vi "2020_day06.vi"() -> ()   [LabVIEW 2021]
panel:
  out "Task 2":i32
  out "Task 1":i32
  in  "Switch":bool caption="Ex. Data  vs.  User Data"
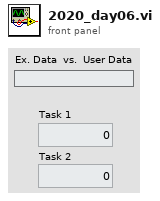
[diagram p1: front panel]
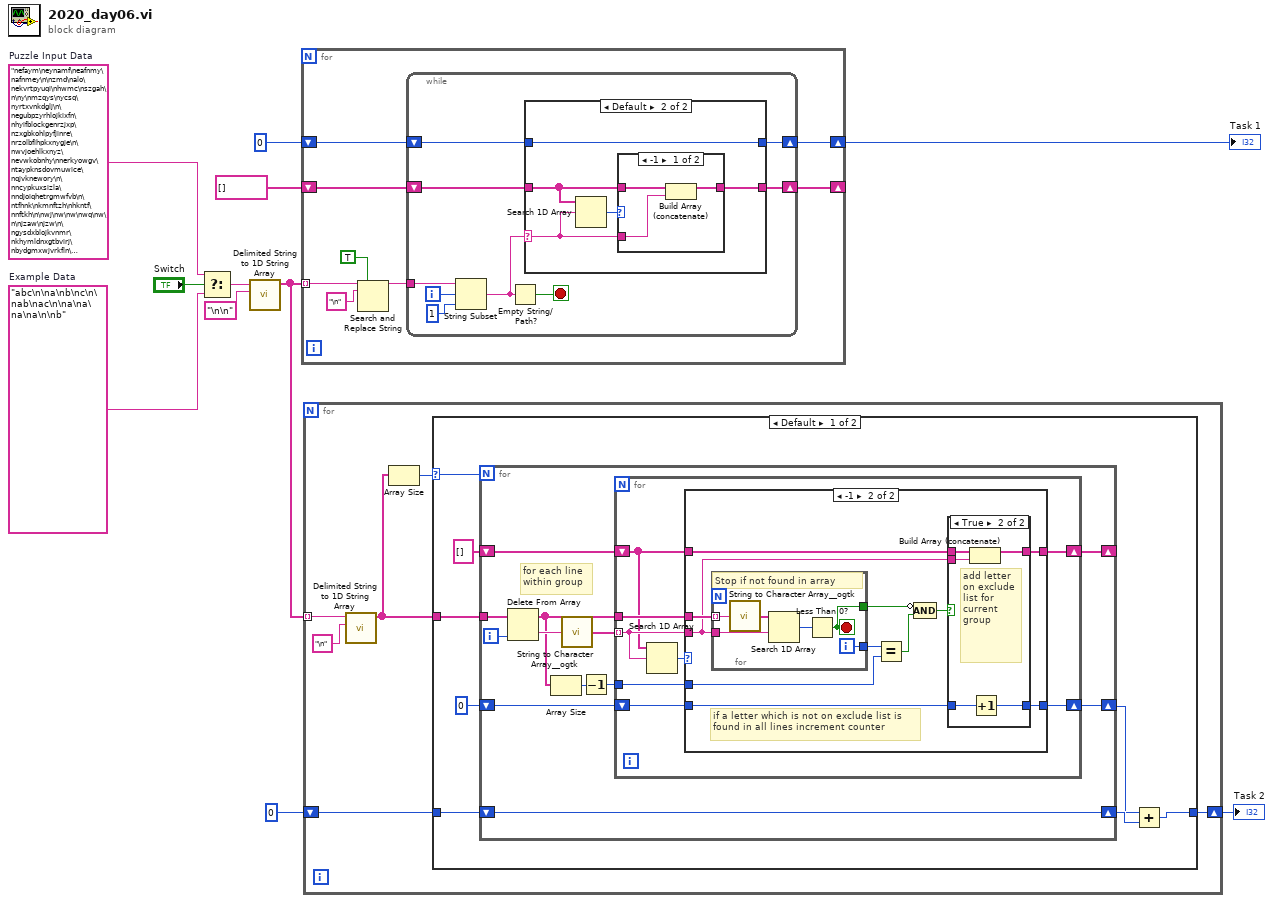
[diagram p0: block diagram]
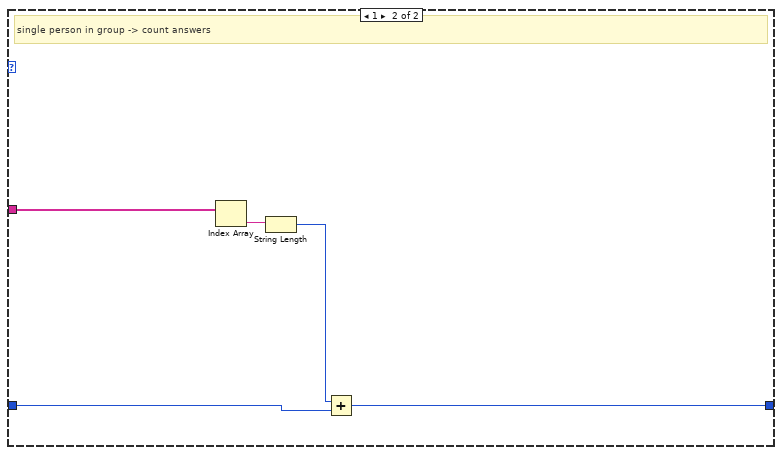
[diagram p4: hidden frame]
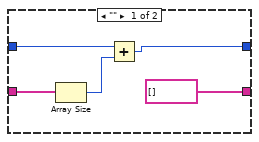
[diagram p5: hidden frame]
diagram:
  w9 = "nefaym\neynamf\neafnmy\nafnmey\n\nzmd\nalo\nekvrtpyuqi\nhwmc\nszgah\n\ny\nmzqys\nycsq\nyrtxvnkdglj\n\negubpzyrhlojkixfn\nhyifblockgenrzjxp\nzxgbkohlpyfjinre\nrzolbfihpkxnygje\n\nwvjoehlkxnyz\nevwkobnhy\nnerkyowgv\ntaypknsdovmuwice\nqjvknewory\n\nncypkuxsizla\nndjoiqhetrgmwfvb\n\ntfhnk\nkmnftzh\nhkntf\nnftkh\n\nwj\nw\nw\nwq\nw\n\njzaw\njzw\n\ngysdxblojkvnmr\nkhymldnxgtbvirj\nbydgmxwjvrkfln\nlykvumdnrxbjg\n\nxce\nxec\nxec\ncex\n\nlacbwdzjofymieug\nqpbhtnywsluirgjaxkfm\n\norzpamlyckgwhjidnq\nmyeqhzijgkdoxwprcvbt\ngzaocylrwkiumpfjqdh\ncqhzpwiyrmkdgjso\n\nd\nvd\nsgohd\n\nr\nr\n\nknyrgtba\ngatbyoknr\nakmgyntbr\narykgnbot\nanyrgbkt\n\niohn\ncoangpuj\non\nknqoi\ntoink\n\nhvramnt\ng..."  # Puzzle Input Data
  w10 = "abc\n\na\nb\nc\n\nab\nac\n\na\na\na\na\n\nb"  # Example Data
  n1 = Select(t=w9, s="Switch", f=w10) -> (s? t:f=w4:string)
  n2 = call <vilib>:"Delimited String to 1D String Array.vi"("delimiter"="\n\n", "delimited string"=w4) -> ("string array"=w1:string[])  [unwired: 9 in]
  n3 = for {
    tunnel: w1 -> [w15] mode=indexing
    shift-right: [w18] -> _
    shift-left: string[] [] ("array type (2D Dbl)") -> [w19]
    shift-right: [w16] -> w6
    shift-left: 0 -> [w17]
    n4 = Search and Replace String(replace all?=TRUE ("replace all? (F)"), input string=w15, search string="\n" ("delimiter")) -> (result string=w14:string)  [unwired: 5 in, 3 out]
    n5 = while {
      tunnel: w14 -> [w27]
      shift-right: [w22] -> w18
      shift-left: w19 -> [w28]
      shift-right: [w20] -> w16
      shift-left: w17 -> [w21]
      i -> [w26]
      stop <- w24 stop-if-true
      n6 = String Subset(string=w27, offset (0)=w26, length (rest)=1 ("length (rest)")) -> (substring=w23:string)
      n7 = Empty String/Path?(string/path=w23) -> (empty?=w24:bool)
      n8 = case shown="Default" w23 {
        selector: w23 -> [_ w35]
        tunnel: w28 -> [w30 w38]
        tunnel: [string[] [] ("array type (2D Dbl)") w37] -> w22
        tunnel: w21 -> [w32 w34]
        tunnel: [w31 w34] -> w20
        frame "" {
          n9 = Array Size(array=w30) -> (size(s)=w33:i32)
          n10 = Add(x=w32, y=w33) -> (x+y=w31:i32)
        }
        frame Default {
          n11 = Search 1D Array(1D array=w38, element=w35) -> (index of element=w36:i32)  [unwired: 1 in]
          n12 = case shown="-1" w36 {
            tunnel: w38 -> [w41 w42]
            tunnel: [w40 w42] -> w37
            tunnel: w35 -> [w39 _]
            frame -1 {
              n13 = Build Array (concatenate)(w41, w39) -> (w40:string[])
            }
            frame Default {
            }
          }
        }
      }
    }
  }
  "Task 1" <- w6
  n14 = for {
    tunnel: w1 -> [w48] mode=indexing
    shift-right: [w43] -> w2
    shift-left: 0 -> [w44]
    n15 = call <vilib>:"Delimited String to 1D String Array.vi"("delimiter"="\n", "delimited string"=w48) -> ("string array"=w45:string[])  [unwired: 9 in]
    n16 = Array Size(array=w45) -> (size(s)=w46:i32)
    n17 = case shown="Default" w46 {
      selector: w46 -> [w53 _]
      tunnel: w45 -> [w56 w106]
      tunnel: [w50 w104] -> w43
      tunnel: w44 -> [w55 w107]
      frame Default {
        n18 = for {
          N: w53 -> [_]
          shift-right: [w64] -> w54
          shift-left: w55 -> [w64]
          tunnel: w56 -> [w58]
          shift-right: [w61] -> _
          shift-left: string[] [] ("array type (2D Dbl)") -> [w62]
          shift-right: [w59] -> w49
          shift-left: 0 -> [w60]
          i -> [w68]
          # "for each line\nwithin group"
          n19 = Delete From Array(array=w58, index=w68) -> (deleted portion=w67:string, array with subset deleted=w57:string[])  [unwired: 1 in]
          n20 = Array Size(array=w57) -> (size(s)=w65:i32)
          n21 = call <userlib>:"String to Character Array__ogtk.vi"("Input String"=w67) -> ("Character Array"=w66:string[])
          n22 = Decrement(x=w65) -> (x-1=w63:i32)
          n23 = for {
            tunnel: w66 -> [w70] mode=indexing
            tunnel: w57 -> [w72]
            shift-right: [w76] -> w59
            shift-left: w60 -> [w74]
            tunnel: w63 -> [w75]
            shift-right: [w71] -> w61
            shift-left: w62 -> [w69]
            n24 = Search 1D Array(1D array=w69, element=w70) -> (index of element=w73:i32)  [unwired: 1 in]
            n25 = case shown="-1" w73 {
              tunnel: w72 -> [_ w89]
              tunnel: w70 -> [_ w82]
              tunnel: [w77 w85] -> w76
              tunnel: w75 -> [_ w87]
              tunnel: w74 -> [w77 w86]
              tunnel: [w78 w84] -> w71
              tunnel: w69 -> [w78 w83]
              frame Default {
              }
              frame -1 {
                # "if a letter which is not on exclude list is found in all lines increment counter"
                n26 = for {
                  tunnel: w89 -> [w102] mode=indexing
                  tunnel: w82 -> [w100]
                  tunnel: [w98] -> w88
                  tunnel: [w97] -> w80
                  i -> [w98]
                  stop <- w97 stop-if-true
                  # "Stop if not found in array"
                  n27 = call <userlib>:"String to Character Array__ogtk.vi"("Input String"=w102) -> ("Character Array"=w101:string[])
                  n28 = Search 1D Array(1D array=w101, element=w100) -> (index of element=w99:i32)  [unwired: 1 in]
                  n29 = Less Than 0?(x=w99) -> (x < 0?=w97:bool)
                }
                n30 = Equal?(x=w88, y=w87) -> (x = y?=w81:bool)
                n31 = Compound Arithmetic op=AND(invert w80, w81) -> (w79:bool)
                n32 = case shown="True" w79 {
                  tunnel: w86 -> [w91 w96]
                  tunnel: [w91 w95] -> w85
                  tunnel: [w90 w93] -> w84
                  tunnel: w83 -> [w90 w94]
                  tunnel: w82 -> [_ w92]
                  frame False {
                  }
                  frame True {
                    # "add letter on exclude list for current group"
                    n33 = Build Array (concatenate)(w94, w92) -> (w93:string[])
                    n34 = Increment(x=w96) -> (x+1=w95:i32)
                  }
                }
              }
            }
          }
        }
        n35 = Add(x=w49, y=w54) -> (x+y=w50:i32)
      }
      frame 1 {
        # "single person in group -> count answers"
        n36 = Index Array(array=w106) -> (element=w105:string)  [unwired: 1 in]
        n37 = String Length(string=w105) -> (length=w103:i32)
        n38 = Add(x=w103, y=w107) -> (x+y=w104:i32)
      }
    }
  }
  "Task 2" <- w2
